vi "ziZoomFFT.vi"(0 "State Input":T6, 1 "Filter Settings":cluster{"Timeconstant (s)":dbl, "Order (#)":i32}={"Timeconstant (s)"=0.0099, "Order (#)"=0} {"Timeconstant (s)" format="%#_3p"}, 2 "Averaging Parameters":T4, 3 "Window (Hanning)":T2=1 items=["Rectangle"=0, "Hanning"=1, "Hamming"=2, "Blackman-Harris"=3, "Exact Blackman"=4, "Blackman"=5, "Flat Top"=6, "4 Term B-Harris "=7, "7 Term B-Harris"=8, "Low Sidelobe"=9, "Blackman Nuttall"=11, "Triangle"=30, "Bartlett-Hanning"=31, "Bohman"=32, "Parzen"=33, "Welch"=34, "Kaiser"=60, "Dolph-Chebyshev"=61, "Gaussian"=62], 5 "Mode (Cont)":T8(ring), 7 "Demod Sample":T7 {"Aux In 1 (V)" format="%#_5p"; "Aux In 0 (V)" format="%#_5p"; "X (Vrms)" format="%#_5p"; "Y (Vrms)" format="%#_5p"; "Osc Phase (rad)" format="%#.3g"}, 9 "Size (512)":i32=512, 10 "clockbase (1/s) (210M=HF2)":dbl=210000000.0 format="%#_6p", 11 "Result Unit":T3(ring), 12 "Log/Linear":enum16{"Linear", "dB", "dBm"}(ring)=enum."dB", 13 "Fitler Compensation (F)":bool) -> (4 "State Output":T5, 6 "Spectra":cluster{"Freqs (Hz)":dbl[], dbl[]}[](array[cluster]), 8 "New FFT":bool, 14 "Averaging Done":bool, 15 "Parameters Out":T1)   [LabVIEW 2009, in "Zurich Instruments LabOne.lvlib"]
doc: "Compute the FFT of the demodulated signal.\n\nUse shift registers for <B>State Input</B> and <B>State Output</B>. <B>New FFT</B> indicates that Spectra and <B>Parameters out</B> contain new data and sample accumulation for a new FFT has begun.\n\n<B>Window</B> The default and recommended window function is the Hanning window. Only change this if you know what you are doing.\n<B>Spectral SNR</B> The peak power spectral density divided by the noise power density.\n<B>SNR</B> The power in the singal band divided by the noise power in the equivalent bandwidth."
uses:
  <instrlib>/Zurich Instruments LabOne/Zurich Instruments LabOne.lvlib
  <instrlib>/Zurich Instruments LabOne/Public/Data/ziTypeDemodSampleEx.ctl
  <vilib>/Analysis/4window.llb/windowTd.ctl
  <vilib>/Analysis/0measdsp.llb/Scaled Time Domain Window (CDB).vi
  <vilib>/measure/maspectr.llb/FFT Power Spectrum for 1 Chan (CDB).vi
  <vilib>/measure/NI_MAPro.lvlib
  <vilib>/Analysis/NI_AALPro.lvlib
panel:
  out "Noise Report":cluster{"Freqs (Hz)":dbl[], "magnitude":dbl[]}[](graph)
  out "Freqs (Hz)":dbl[](array[numeric])
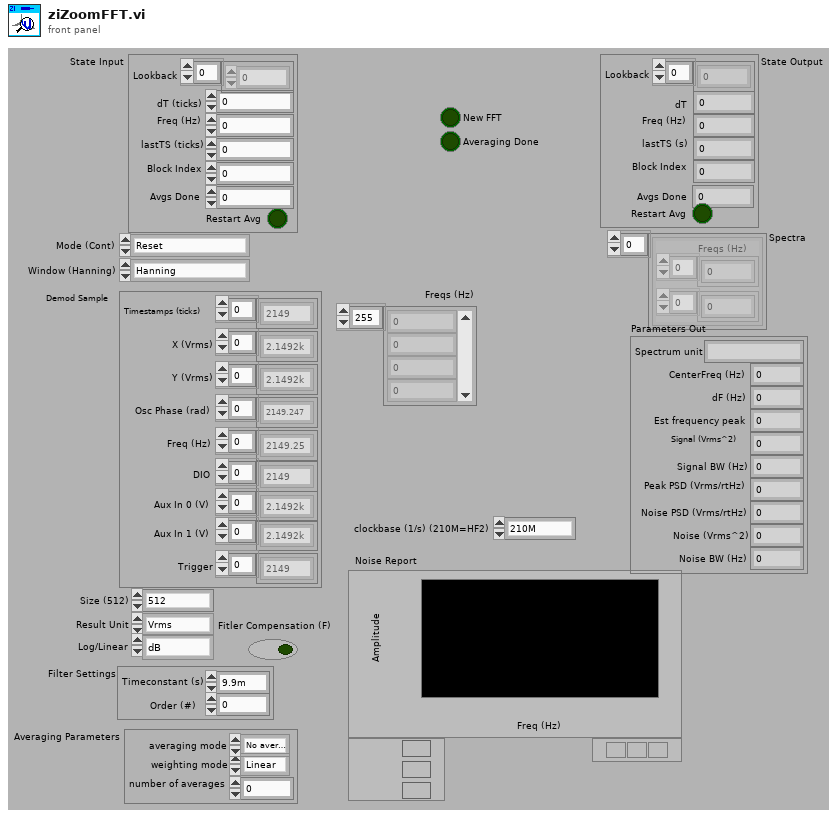
[diagram p1: front panel]
types:
  T1 = cluster{"Spectrum unit":string, "CenterFreq (Hz)":dbl, "dF (Hz)":dbl, "Est frequency peak":dbl, "Signal (Vrms^2)":dbl, "Signal BW (Hz)":dbl, "Peak PSD (Vrms/rtHz)":dbl, "Noise PSD (Vrms/rtHz)":dbl, "Noise (Vrms^2)":dbl, "Noise BW (Hz)":dbl}
  T2 = typedef "NI_AALPro.lvlib/windowTd.ctl" = u32
  T3 = enum32{"Vrms", "Vpk", "Vrms^2", "Vpk^2", "Vrms/rtHz", "Vpk/rtHz", "Vrms^2/Hz", "Vpk^2/Hz"}
  T4 = cluster{"averaging mode":enum16{"No averaging", "Vector averaging", "RMS averaging", "Peak hold"}, "weighting mode":enum16{"Linear", "Exponential"}, "number of averages":u32}
  T5 = cluster{"Lookback":cdb[], "dT":u64, "Freq (Hz)":dbl, "lastTS (s)":u64, "Block Index":i32, "Avgs Done":i32, "Restart Avg":bool}
  T6 = cluster{"Lookback":cdb[], "dT (ticks)":u64, "Freq (Hz)":dbl, "lastTS (ticks)":u64, "Block Index":i32, "Avgs Done":i32, "Restart Avg":bool}
  T7 = typedef "ziTypeDemodSampleEx.ctl" = cluster{"Timestamps (ticks)":u64[], "X (Vrms)":dbl[], "Y (Vrms)":dbl[], "Osc Phase (rad)":dbl[], "Freq (Hz)":dbl[], "DIO":u32[], "Aux In 0 (V)":dbl[], "Aux In 1 (V)":dbl[], "Trigger":u32[]}
  T8 = enum16{"Reset", "Data block wise", "Data continuous", "Data cont calc"}
  T9 = enum16{"Reset", "Data Block Wise", "Data Continuous", "Calculate Continuous", "Settings"}
  T10 = enum16{"Power (Vrms^2)", "Amplitude (Vrms)", "Gain (amplitude ratio)"}
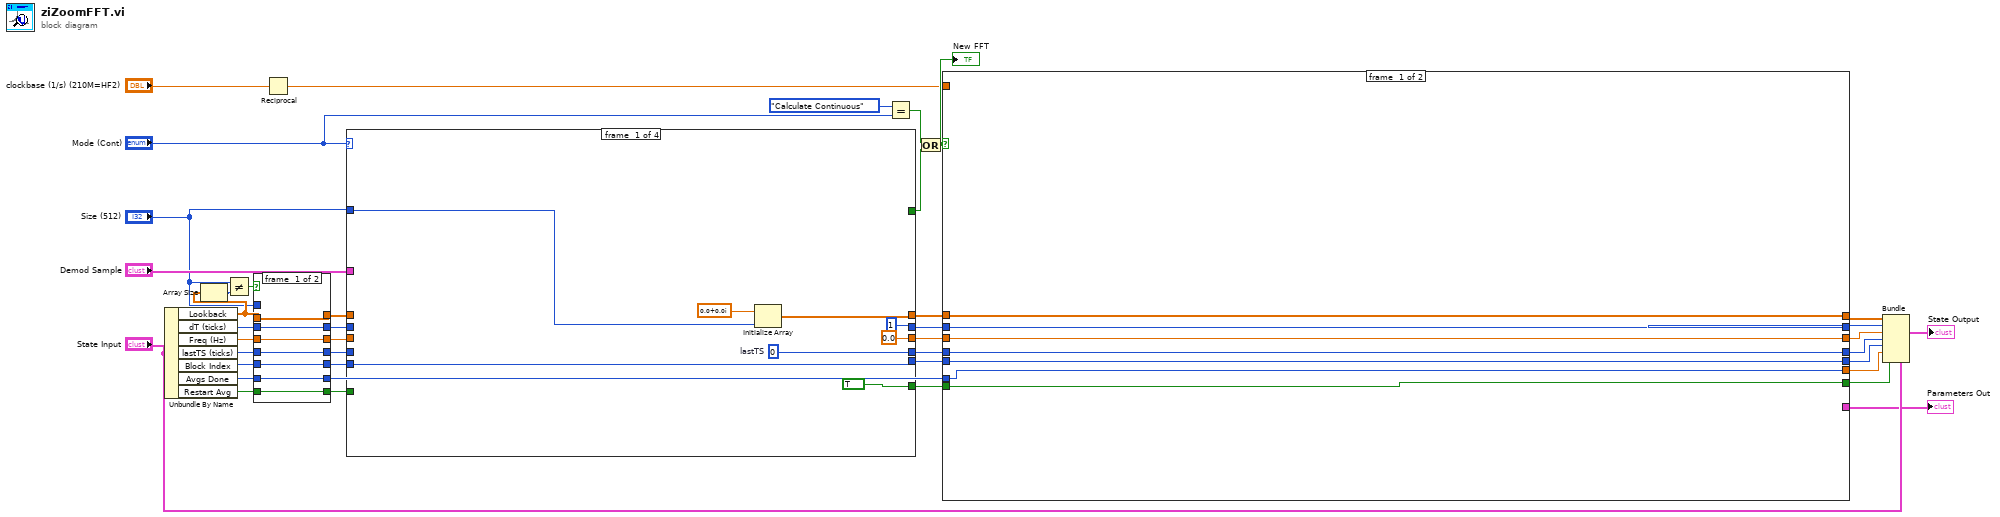
[diagram p0: block diagram]
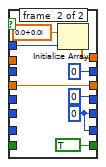
[diagram p2: hidden frame]
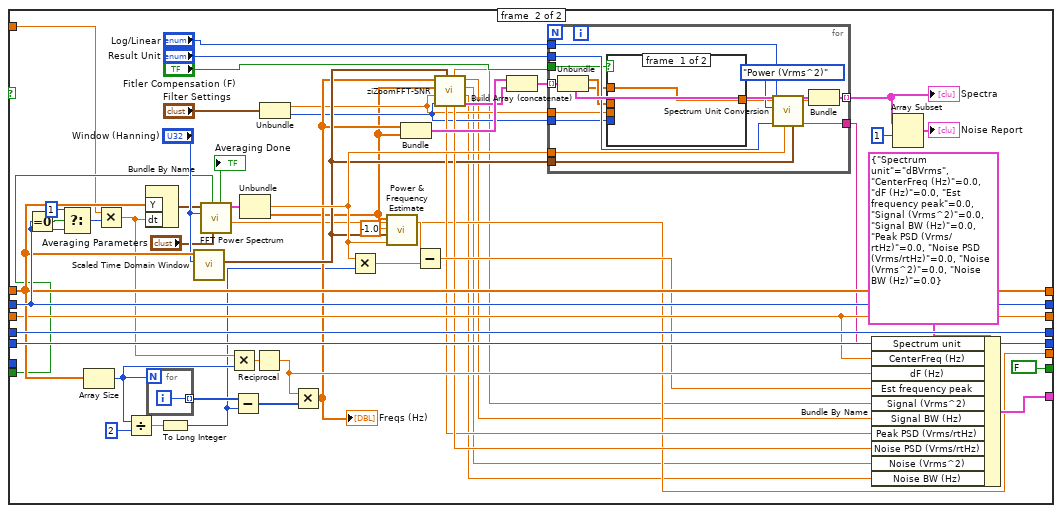
[diagram p3: hidden frame]
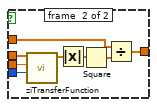
[diagram p4: hidden frame]
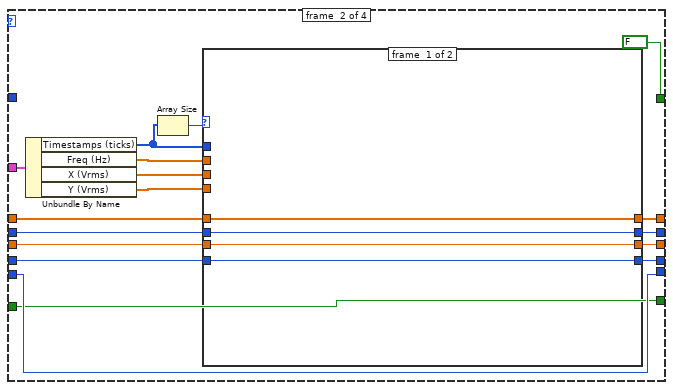
[diagram p5: hidden frame]
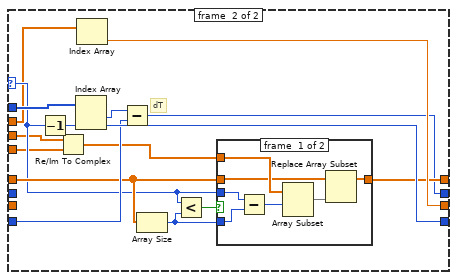
[diagram p6: hidden frame]
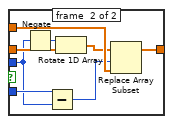
[diagram p7: hidden frame]
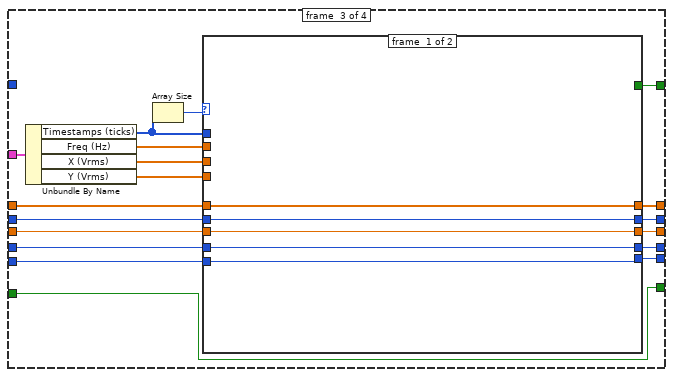
[diagram p8: hidden frame]
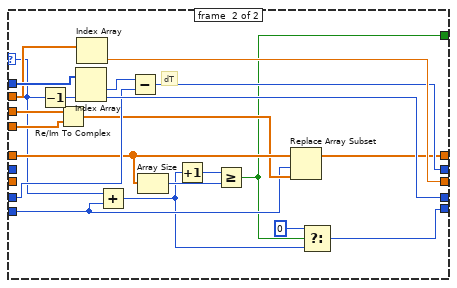
[diagram p9: hidden frame]
diagram:
  n1 = Unbundle By Name("State Input") -> ("Lookback"=w21:cdb[], "dT (ticks)"=w18:u64, "Freq (Hz)"=w17:dbl, "lastTS (ticks)"=w16:u64, "Block Index"=w15:i32, "Avgs Done"=w9:i32, "Restart Avg"=w6:bool)
  n2 = Array Size(array=w21) -> (size(s)=w23:i32)
  n3 = Not Equal?(x="Size (512)", y=w23) -> (x != y?=w22:bool)
  n4 = case shown="True" w22 {
    tunnel: "Size (512)" -> [_ w55]
    tunnel: w21 -> [w48 _]
    tunnel: [w48 w54] -> w19
    tunnel: w18 -> [w44 _]
    tunnel: w17 -> [w45 w51]
    tunnel: w16 -> [w46 _]
    tunnel: w15 -> [w47 _]
    tunnel: [w47 w50] -> w14
    tunnel: [w46 u64 0 ("lastTS (s)")] -> w13
    tunnel: [w45 w51] -> w12
    tunnel: [w44 u64 0 ("dT")] -> w11
    tunnel: w9 -> [w43 _]
    tunnel: [w43 w50] -> w8
    tunnel: w6 -> [w42 _]
    tunnel: [w42 TRUE ("Restart Avg")] -> w5
    frame #0 {
    }
    frame #1 {
      w50 = 0 ("Block Index")
      n5 = Initialize Array(cdb 0.0+0.0i ("element"), w55) -> (w54:cdb[])
    }
  }
  n6 = Reciprocal(x="clockbase (1/s) (210M=HF2)") -> (1/x=w1:dbl)
  n7 = case shown="\"Data continuous\", \"Data cont calc\"" "Mode (Cont)" {
    tunnel: w19 -> [_ w76 w129 w166]
    tunnel: [w63 w72 w125 w166] -> w38
    tunnel: "Demod Sample" -> [_ w81 w134 _]
    tunnel: w13 -> [_ w78 w131 w163]
    tunnel: [w62 w77 w130 w163] -> w35
    tunnel: w12 -> [_ w70 w123 w164]
    tunnel: [0.0 ("Freq (Hz)") w71 w124 w164] -> w36
    tunnel: w11 -> [_ w69 w122 w165]
    tunnel: [u64 1 w68 w121 w165] -> w37
    tunnel: w14 -> [w59 w67 w120 w162]
    tunnel: [w59 w67 w119 w162] -> w34
    tunnel: [_ FALSE w118 _] -> w28
    tunnel: "Size (512)" -> [w58 _ _ _]
    tunnel: [TRUE ("averaging done") w65 w117 w161] -> w10
    tunnel: w5 -> [_ w65 w117 w161]
    frame #0 {
      w62 = u64 0  # lastTS
      n8 = Initialize Array(cdb 0.0+0.0i ("element"), w58) -> (w63:cdb[])
    }
    frame #1 {
      n9 = Unbundle By Name(w81) -> ("Timestamps (ticks)"=w79:u64[], "Freq (Hz)"=w73:dbl[], "X (Vrms)"=w75:dbl[], "Y (Vrms)"=w74:dbl[])
      n10 = Array Size(array=w79) -> (size(s)=w80:i32)
      n11 = case shown="Default" w80 {
        selector: w80 -> [_ w94]
        tunnel: w79 -> [_ w101]
        tunnel: w78 -> [w82 w97]
        tunnel: [w82 w99] -> w77
        tunnel: w76 -> [w85 w96]
        tunnel: w75 -> [_ w92]
        tunnel: w74 -> [_ w91]
        tunnel: w73 -> [_ w89]
        tunnel: [w85 w87] -> w72
        tunnel: [w84 w88] -> w71
        tunnel: w70 -> [w84 _]
        tunnel: w69 -> [w83 _]
        tunnel: [w83 w86] -> w68
        frame #0 {
        }
        frame #1 {
          # "dT"
          n12 = Decrement(x=w94) -> (x-1=w100:i32)
          n13 = Re/Im To Complex(1:w91, 2:w92) -> (0:w90:cdb[])
          n14 = Index Array(array=w101, index #2=w100) -> (element #1=w98:u64, element #2=w99:u64)  [unwired: 1 in]
          n15 = Index Array(array=w89) -> (element=w88:dbl)  [unwired: 1 in]
          n16 = Subtract(x=w98, y=w97) -> (x-y=w86:u64)
          n17 = Array Size(array=w96) -> (size(s)=w93:i32)
          n18 = Less?(x=w94, y=w93) -> (x < y?=w95:bool)
          n19 = case shown="True" w95 {
            tunnel: w90 -> [w106 w116]
            tunnel: [w102 w109] -> w87
            tunnel: w94 -> [w108 w112]
            tunnel: w96 -> [w103 w113]
            tunnel: w93 -> [w107 w115]
            frame #0 {
              n20 = Subtract(x=w108, y=w107) -> (x-y=w105:i32)
              n21 = Array Subset(array=w106, index=w105) -> (w104:cdb[])  [unwired: 1 in]
              n22 = Replace Array Subset(array=w103, new element=w104) -> (w102:cdb[])  [unwired: 1 in]
            }
            frame #1 {
              n23 = Negate(x=w112) -> (-x=w110:i32)
              n24 = Subtract(x=w115, y=w112) -> (x-y=w114:i32)
              n25 = Rotate 1D Array(1:w113, 2:w110) -> (0:w111:cdb[])
              n26 = Replace Array Subset(array=w111, new element=w116, index=w114) -> (w109:cdb[])
            }
          }
        }
      }
    }
    frame #2 {
      n27 = Unbundle By Name(w134) -> ("Timestamps (ticks)"=w132:u64[], "Freq (Hz)"=w126:dbl[], "X (Vrms)"=w128:dbl[], "Y (Vrms)"=w127:dbl[])
      n28 = Array Size(array=w132) -> (size(s)=w133:i32)
      n29 = case shown="Default" w133 {
        selector: w133 -> [_ w147]
        tunnel: w132 -> [_ w160]
        tunnel: w131 -> [w136 w156]
        tunnel: [w136 w158] -> w130
        tunnel: w129 -> [w139 w155]
        tunnel: w128 -> [_ w154]
        tunnel: w127 -> [_ w153]
        tunnel: w126 -> [_ w151]
        tunnel: [w139 w148] -> w125
        tunnel: [w138 w150] -> w124
        tunnel: w123 -> [w138 _]
        tunnel: w122 -> [w137 _]
        tunnel: [w137 w149] -> w121
        tunnel: w120 -> [w135 w146]
        tunnel: [w135 w140] -> w119
        tunnel: [_ w142] -> w118
        frame #0 {
        }
        frame #1 {
          # "dT"
          n30 = Decrement(x=w147) -> (x-1=w159:i32)
          n31 = Re/Im To Complex(1:w153, 2:w154) -> (0:w152:cdb[])
          n32 = Index Array(array=w160, index #2=w159) -> (element #1=w157:u64, element #2=w158:u64)  [unwired: 1 in]
          n33 = Index Array(array=w151) -> (element=w150:dbl)  [unwired: 1 in]
          n34 = Add(x=w147, y=w146) -> (x+y=w143:i32)
          n35 = Subtract(x=w157, y=w156) -> (x-y=w149:u64)
          n36 = Array Size(array=w155) -> (size(s)=w145:i32)
          n37 = Increment(x=w143) -> (x+1=w144:i32)
          n38 = Greater Or Equal?(x=w144, y=w145) -> (x >= y?=w142:bool)
          n39 = Replace Array Subset(array=w155, new element=w152, index=w146) -> (w148:cdb[])
          n40 = Select(t=0, s=w142, f=w143) -> (s? t:f=w140:i32)
        }
      }
    }
    frame #3 {
    }
  }
  n41 = Equal?(x=T9."Calculate Continuous", y="Mode (Cont)") -> (x = y?=w27:bool)
  n42 = Or(x=w27, y=w28) -> (x .or. y?=w24:bool)
  "New FFT" <- w24
  n43 = case shown="True" w24 {
    tunnel: w38 -> [w173 w217]
    tunnel: w37 -> [w172 w218]
    tunnel: w36 -> [w171 w214]
    tunnel: w35 -> [w170 w223]
    tunnel: w34 -> [w169 w222]
    tunnel: [w173 w217] -> w33
    tunnel: [w172 w218] -> w32
    tunnel: [w171 w214] -> w31
    tunnel: [w170 w223] -> w30
    tunnel: [w169 w222] -> w29
    tunnel: [_ w213] -> w3
    tunnel: w10 -> [w167 w185]
    tunnel: w8 -> [w168 _]
    tunnel: [w168 w184] -> w7
    tunnel: [w167 FALSE ("averaging done")] -> w4
    tunnel: w1 -> [_ w176]
    frame #0 {
    }
    frame #1 {
      n44 = Equal To 0?(x=w218) -> (x = 0?=w219:bool)
      n45 = Select(t=u64 1, s=w219, f=w218) -> (s? t:f=w178:u64)
      n46 = Array Size(array=w217) -> (size(s)=w224:i32)
      n47 = Multiply(x=w176, y=w178) -> (x*y=w177:dbl)
      n48 = Divide(x=w224, y=2) -> (x/y=w211:dbl)
      n49 = Bundle By Name("Y"=w217, "dt"=w177) -> (w197:waveform(cdb))  [unwired: 1 in]
      n50 = for {
        N: w224 -> [_]
        tunnel: [w253] -> w228 mode=indexing
        i -> [w253]
      }
      n51 = To Long Integer(number=w211) -> (32bit integer=w174:i32)
      n52 = call-poly <vilib>:"Scaled Time Domain Window.vi"("window"="Window (Hanning)", "X"=w217) -> ("window properties"=w190:cluster{"eq noise BW":dbl, "coherent gain":dbl})  [unwired: 7 in, 2 out]
      n53 = call-poly <vilib>:"FFT Power Spectrum.vi"("averaging parameters"="Averaging Parameters", "restart averaging (F)"=w185, "window"="Window (Hanning)", "time signal"=w197) -> ("averages completed"=w184:dbl, "power spectrum"=w196:cluster{"f0":dbl, "df":dbl, "magnitude":dbl[]}, "averaging done"=→"Averaging Done":bool)  [unwired: 4 in, 1 out]
      n54 = Multiply(x=w177, y=w224) -> (x*y=w225:dbl)
      n55 = Subtract(x=w228, y=w174) -> (x-y=w226:i32[])
      n56 = Unbundle(w196) -> ("df"=w201:dbl, "magnitude"=w175:dbl[])  [unwired: 1 out]
      n57 = Reciprocal(x=w225) -> (1/x=w215:dbl)
      n58 = Unbundle("Filter Settings") -> ("Timeconstant (s)"=w187:dbl, "Order (#)"=w188:i32)
      n59 = Multiply(x=w215, y=w226) -> (x*y=w189:dbl[])
      "Freqs (Hz)" <- w189
      n60 = Multiply(x=w201, y=w174) -> (x*y=w210:dbl)
      n61 = call <vilib>:"Power & Frequency Estimate.vi"("df"=w201, "window constants"=w190, "peak frequency (max)"=-1.0, "Power Spectrum (V^2 rms)"=w175) -> ("est frequency peak"=w209:dbl)  [unwired: 2 in, 1 out]
      n62 = Bundle(w189, "magnitude"=w175) -> (w204:cluster{dbl[], "magnitude":dbl[]})  [unwired: 1 in]
      n63 = Subtract(x=w209, y=w210) -> (x-y=w208:dbl)
      n64 = call <instrlib>:"ziZoomFFT-SNR.vi"("window properties"=w190, "Order (#)"=w188, "Timeconstant (s)"=w187, "Powerspectrum (Vrms^2)"=w175, "Freqs (Hz)"=w189) -> ("Segmentation"=w194:cluster{"Freqs (Hz)":dbl[], dbl[]}[], "Noise BW (Hz)"=w179:dbl, "Noise (Vrms^2)"=w180:dbl, "Signal BW (Hz)"=w181:dbl, "Noise PSD (Vrms/rtHz)"=w192:dbl, "Signal (Vrms^2)"=w182:dbl, "Peak PSD (Vrms/rtHz)"=w191:dbl)
      n65 = Build Array (concatenate)(w204, w194) -> (w203:cluster{"Freqs (Hz)":dbl[], "magnitude":dbl[]}[])
      n66 = for {
        tunnel: w203 -> [w243] mode=indexing
        tunnel: [w241] -> w200 mode=indexing
        tunnel: "Log/Linear" -> [w239]
        tunnel: "Result Unit" -> [w238]
        tunnel: [w237] -> w202
        tunnel: w190 -> [w236]
        tunnel: w201 -> [w231]
        tunnel: w188 -> [w234]
        tunnel: w187 -> [w233]
        tunnel: "Fitler Compensation (F)" -> [w232]
        n67 = Unbundle(w243) -> ("Freqs (Hz)"=w235:dbl[], "magnitude"=w230:dbl[])
        n68 = case shown="True" w232 {
          tunnel: w230 -> [w244 w251]
          tunnel: [w244 w250] -> w229
          tunnel: w235 -> [_ w245]
          tunnel: w233 -> [_ w252]
          tunnel: w234 -> [_ w246]
          frame #0 {
          }
          frame #1 {
            n69 = call <instrlib>:"ziTransferFunction.vi"("Order (#)"=w246, "Timeconstant (s)"=w252, "Frequencies (Hz)"=w245) -> ("TransferFunction"=w249:cdb[])  [unwired: 8 in]
            n70 = Absolute Value(x=w249) -> (abs(x)=w247:dbl[])
            n71 = Square(x=w247) -> (x^2=w248:dbl[])
            n72 = Divide(x=w251, y=w248) -> (x/y=w250:dbl[])
          }
        }
        n73 = call <vilib>:"Spectrum Unit Conversion.vi"("window constants"=w236, "df"=w231, "display unit"=w238, "log/linear"=w239, "spectrum type"=T10."Power (Vrms^2)", "Spectrum in"=w229) -> ("spectrum unit"=w237:string, "Spectrum out"=w242:dbl[])  [unwired: 4 in]
        n74 = Bundle(cluster=w243, "magnitude"=w242) -> (w241:cluster{"Freqs (Hz)":dbl[], "magnitude":dbl[]})  [unwired: 1 in]
      }
      "Spectra" <- w200
      n75 = Bundle By Name(cluster=T1 {"Spectrum unit"="dBVrms", "CenterFreq (Hz)"=0.0, "dF (Hz)"=0.0, "Est frequency peak"=0.0, "Signal (Vrms^2)"=0.0, "Signal BW (Hz)"=0.0, "Peak PSD (Vrms/rtHz)"=0.0, "Noise PSD (Vrms/rtHz)"=0.0, "Noise (Vrms^2)"=0.0, "Noise BW (Hz)"=0.0} ("Parameters out"), "Spectrum unit"=w202, "CenterFreq (Hz)"=w214, "dF (Hz)"=w215, "Est frequency peak"=w208, "Signal (Vrms^2)"=w182, "Signal BW (Hz)"=w181, "Peak PSD (Vrms/rtHz)"=w191, "Noise PSD (Vrms/rtHz)"=w192, "Noise (Vrms^2)"=w180, "Noise BW (Hz)"=w179) -> (w213:T1)
      n76 = Array Subset(array=w200, index=1) -> (→"Noise Report":cluster{"Freqs (Hz)":dbl[], "magnitude":dbl[]}[])  [unwired: 1 in]
    }
  }
  "Parameters Out" <- w3
  n77 = Bundle(cluster="State Input", "Lookback"=w33, "dT (ticks)"=w32, "Freq (Hz)"=w31, "lastTS (ticks)"=w30, "Block Index"=w29, "Avgs Done"=w7, "Restart Avg"=w4) -> (→"State Output":T6)
